vi "get ready status.vi"(0 "Serial Port":refnum<visa-resource-name>) -> (4 "Serial Port":refnum<visa-resource-name>, 6 "ready":bool, 8 "ramp":string, 10 "run status":T1(ring), 15 "Not Ready":T2)   [LabVIEW 2012]
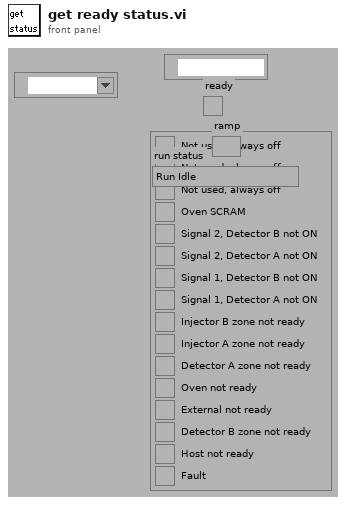
[diagram p1: front panel]
types:
  T1 = enum16{"Run Idle", "Pre Run", "SCC Pre Run 1", "SCC Pre Run 2", "SCC Run", "Run Active", "Report 1", "Report 2", "Run Disabled (from outside GC)"}
  T2 = cluster{"Not used, always off":bool, "Not used, always off":bool, "Not used, always off":bool, "Oven SCRAM":bool, "Signal 2, Detector B not ON":bool, "Signal 2, Detector A not ON":bool, "Signal 1, Detector B not ON":bool, "Signal 1, Detector A not ON":bool, "Injector B zone not ready":bool, "Injector A zone not ready":bool, "Detector A zone not ready":bool, "Oven not ready":bool, "External not ready":bool, "Detector B zone not ready":bool, "Host not ready":bool, "Fault":bool}
  T3 = cluster{"[0]":bool, "[1]":bool, "[2]":bool, "[3]":bool, "[4]":bool, "[5]":bool, "[6]":bool, "[7]":bool, "[8]":bool, "[9]":bool, "[10]":bool, "[11]":bool, "[12]":bool, "[13]":bool, "[14]":bool, "[15]":bool}
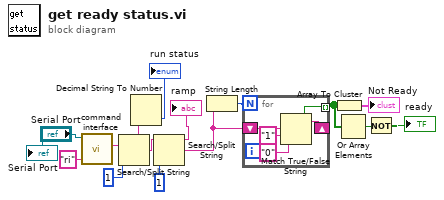
[diagram p0: block diagram]
diagram:
  n1 = call "command interface.vi"("command"="ri", "Serial Port"="Serial Port") -> ("response"=w10:string)  [unwired: 5 in, 3 out]
  n2 = Search/Split String(string=w10, offset (0)=1) -> (substring before match=w12:string, match + rest of string=w13:string)  [unwired: 1 in, 1 out]
  n3 = Decimal String To Number(string=w12) -> (number=→"run status":i32)  [unwired: 2 in, 1 out]
  n4 = Search/Split String(string=w13, offset (0)=1) -> (substring before match=→"ramp":string, match + rest of string=w15:string)  [unwired: 1 in, 1 out]
  n5 = String Length(string=w15) -> (length=w9:i32)
  n6 = for {
    N: w9 -> [_]
    shift-right: [w18] -> _
    shift-left: w15 -> [w17]
    tunnel: [w16] -> w7 mode=indexing
    n7 = Match True/False String(2:"0", 3:"1", 4:w17) -> (0:w16:bool, 1:w18:string)
  }
  n8 = Array To Cluster(array=w7) -> (cluster=→"Not Ready":T3)
  n9 = Or Array Elements(Boolean array=w7) -> (logical OR=w6:bool)
  n10 = Not(x=w6) -> (.not. x?=→"ready":bool)
  "Serial Port" <- "Serial Port"
